vi "Test-Left Motors.vi"() -> ()   [LabVIEW 2014, in "Comp Driver.lvlib"]
uses:
  Comp Driver.lvlib
  Robot Actor Framework/Trace/Trace Controller Class/Config.ctl
  Comp Motors with Encoders/Comp Motors with Encoders Class/Motor Controller Config.ctl
  Robot/Motor with Encoders/Motors with Encoders Class/Motors with Encoders Config.ctl
  Comp Motors with Encoders/Comp Motors with Encoders Class/Encoder Config.ctl
  Comp Trace Controller/Comp Trace Controller Class/Comp Trace Controller.lvclass
  Comp Motors with Encoders/Comp Motors with Encoders Class/Comp Motors with Encoders.lvclass
  Comp Pressure/Comp Pressure Class/Comp Pressure.lvclass
  <vilib>/Rock Robotics/WPI/DriverStation/WPI_DriverStationRobotMode2.ctl
  Robot/Motor with Encoders/Motors with Encoders Messages/Set Rate Msg/Set Rate  (RPM) Msg.lvclass/Set Rate  (RPM) Msg.ctl
  <vilib>/ActorFramework/Message Enqueuer/Message Enqueuer.lvclass/Message Enqueuer.ctl
  <vilib>/ActorFramework/Message Enqueuer/Enqueue.vi
  <vilib>/ActorFramework/Message Priority Queue/Priority Enqueue.vi
  Robot/Motor with Encoders/Motors with Encoders Messages/Set Rate Msg/Set Rate  (RPM) Msg.lvclass
  <vilib>/ActorFramework/Stop Msg/Stop Msg.lvclass
  <vilib>/ActorFramework/Actor/Actor.lvclass
  Robot Actor Framework/Trace/Trace Controller Class/Trace Controller.lvclass
  Robot/Motor with Encoders/Motors with Encoders Class/Motors with Encoders.lvclass
panel:
  in  "Encoder Config":T1={"P"=1.0, "D"=0.0, "F"=0.01, "I"=0.01, "Reverse Feedback Sensor"=FALSE, "Encoder Codes Per Rev"=256}
  out "Enable Tele":bool caption="Enabled Teleop"
  in  "Stop Test Loop 1":bool=TRUE
  in  "Finish Test":bool=TRUE
  in  "Start Test":bool=TRUE
  in  "Rate (RPM)":dbl
  in  "Motos with Encoder Config":T2={"Counts  Per Revolution"=256, "Invert Encoder Direction"=FALSE, "Diameter of Revolution"=6.0, "Max RPM"=0.0, "Encoder Control"=TRUE}
  in  "Slave Motor Controller Configs":T3[](array[typedef])=[{"Device Number"=10, "Invert Motor"=FALSE}]
  in  "Master Motor Controller Config":T3={"Device Number"=9, "Invert Motor"=FALSE}
  in  "Config":T4={"Folder Pattern"="/media/sd%s1", "Starting Letter Position"=1, "Min Free Space (MB)"=50.0, "Max Folders to Check"=10, "Trace Level"=enum."Debug"} {"Min Free Space (MB)" format="%#_13g"}
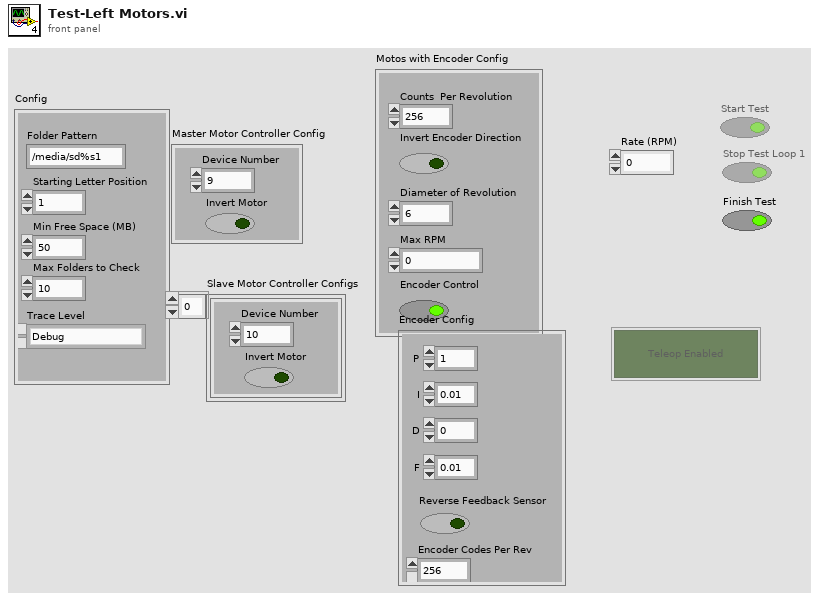
[diagram p1: front panel]
types:
  T1 = typedef "Comp Motors with Encoders.lvlib/Comp Motors with Encoders.lvclass/Encoder Config.ctl" = cluster{"P":dbl, "D":dbl, "F":dbl, "I":dbl, "Reverse Feedback Sensor":bool, "Encoder Codes Per Rev":u16}
  T2 = typedef "Motors with Encoders.lvlib/Motors with Encoders.lvclass/Motors with Encoders Config.ctl" = cluster{"Counts  Per Revolution":u32, "Invert Encoder Direction":bool, "Diameter of Revolution":dbl, "Max RPM":dbl, "Encoder Control":bool}
  T3 = typedef "Comp Motors with Encoders.lvlib/Comp Motors with Encoders.lvclass/Motor Controller Config.ctl" = cluster{"Device Number":u8, "Invert Motor":bool}
  T4 = typedef "Robot Actor Framework.lvlib/Trace.lvlib/Trace Controller.lvclass/Config.ctl" = cluster{"Folder Pattern":string, "Starting Letter Position":i32, "Min Free Space (MB)":dbl, "Max Folders to Check":u32, "Trace Level":enum16{"Critical", "Error", "Warning", "Informational", "Debug"}}
  T5 = enum8{"Enabled", "Disabled", "Disabled and Grayed Out"}
  T6 = enum16{"Critical", "Error", "Warning", "Informational", "Debug"}
  T7 = typedef "WPI_DriverStationRobotMode2.ctl" = enum16{"Autonomous Disabled", "Autonomous Enabled", "Teleop Disabled", "Teleop Enabled", "Disconnected", "Finish", "Test Disabled", "Test Enabled", "Emergency Stopped"}
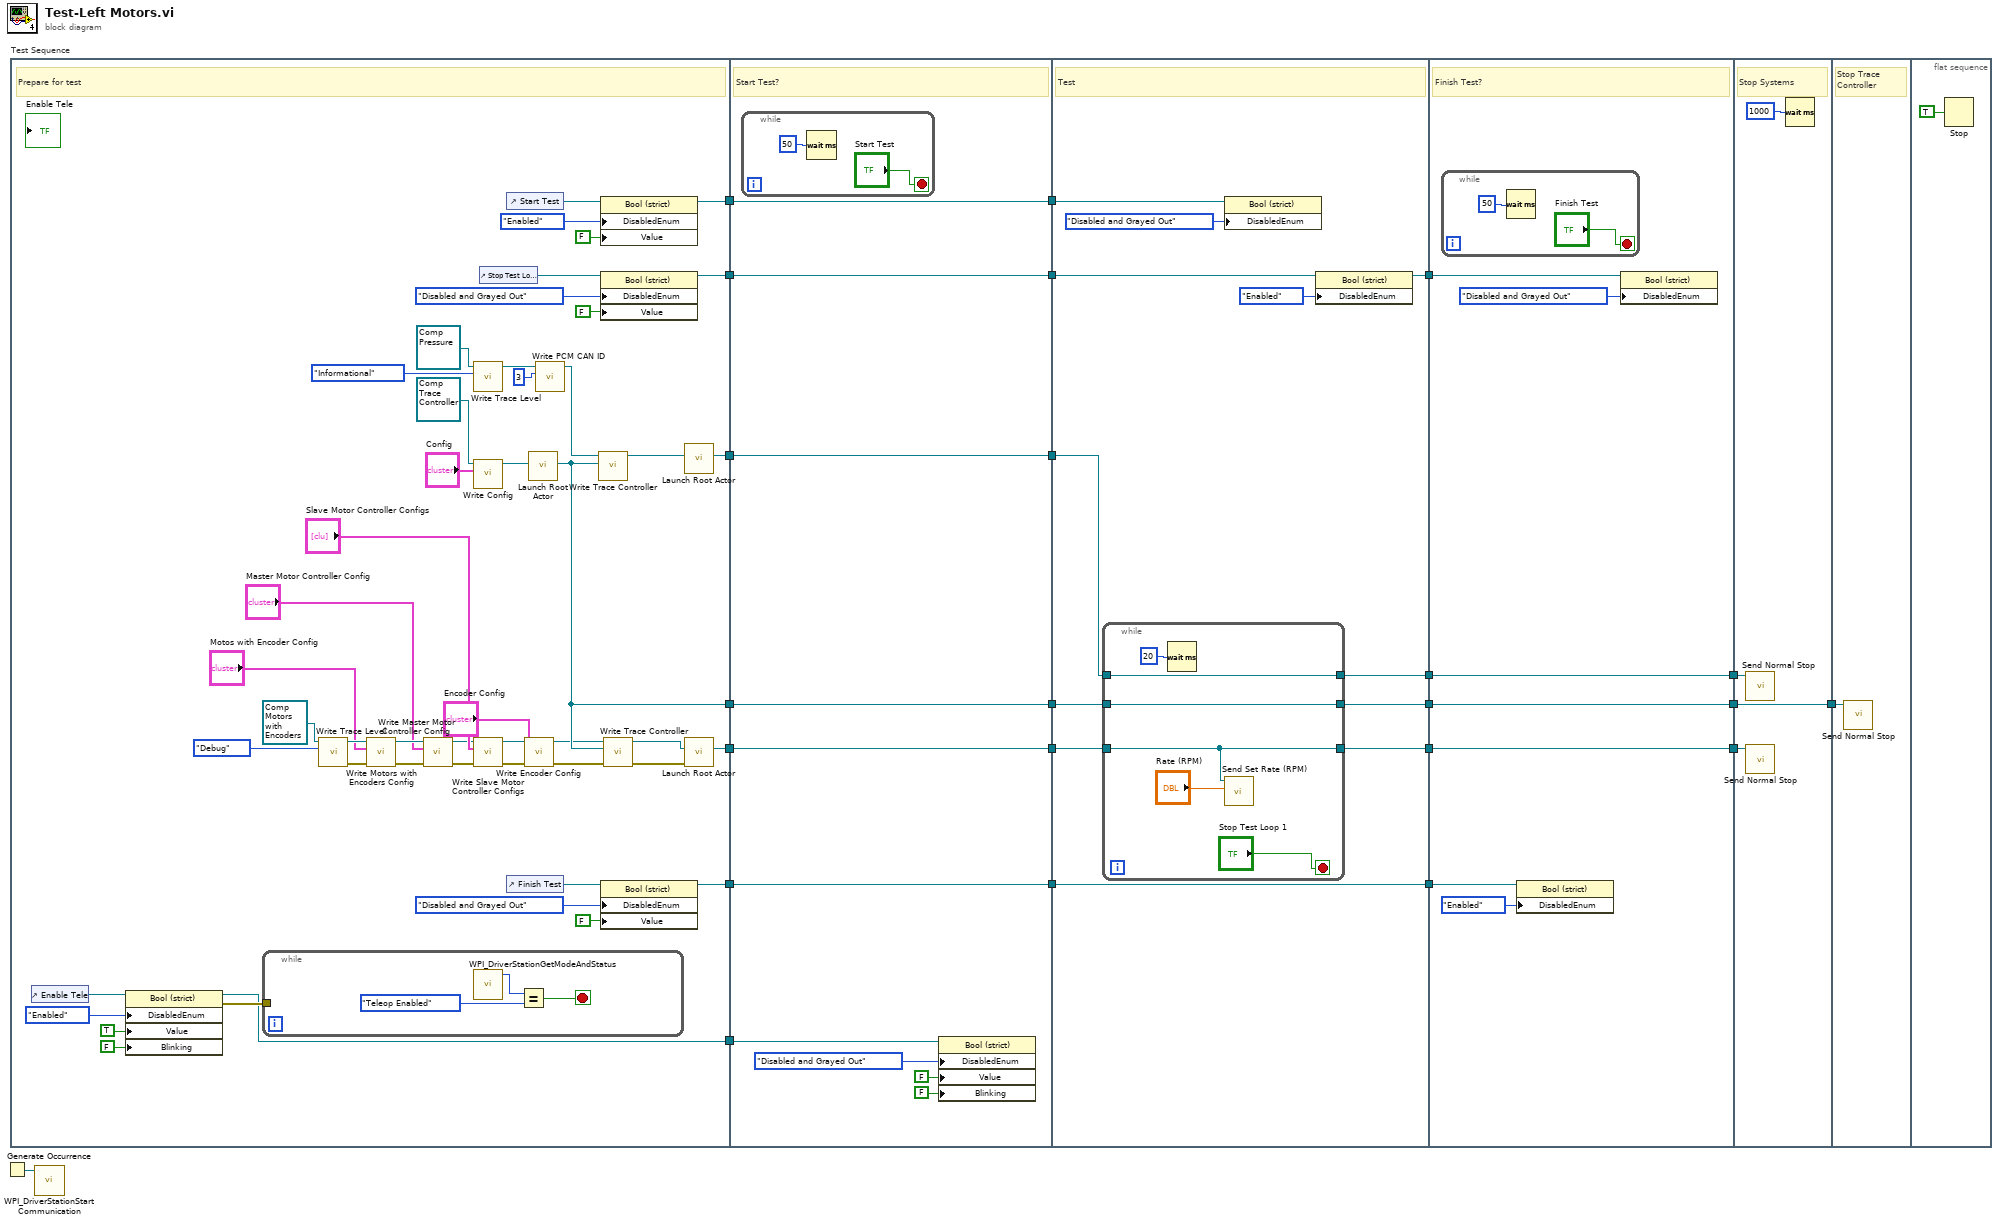
[diagram p0: block diagram]
diagram:
  n1 = Generate Occurrence() -> (w23:refnum<k4>)
  n2 = flat-sequence "Test Sequence" {
    tunnel: [w47] -> w12
    tunnel: [w49] -> w11
    tunnel: [w48] -> w10
    tunnel: [w37] -> w9
    tunnel: [w36] -> w7
    tunnel: [w35] -> w2
    tunnel: [w29] -> w1
    tunnel: [w84] -> w15
    tunnel: [w83] -> w14
    tunnel: [w82] -> w13
    tunnel: w12 -> [w84]
    tunnel: w11 -> [w83]
    tunnel: w10 -> [w82]
    tunnel: w9 -> [w81]
    tunnel: [w81] -> w8
    tunnel: w7 -> [w80]
    tunnel: [w80] -> w6
    tunnel: [w79] -> w3
    tunnel: w2 -> [w79]
    tunnel: w1 -> [w78]
    tunnel: [w93] -> w18
    tunnel: [w95] -> w17
    tunnel: [w94] -> w16
    tunnel: w15 -> [w98]
    tunnel: w14 -> [w96]
    tunnel: w13 -> [w97]
    tunnel: w8 -> [w92]
    tunnel: w6 -> [w90]
    tunnel: [w88] -> w5
    tunnel: [w87] -> w4
    tunnel: w3 -> [w87]
    tunnel: [w111] -> w21
    tunnel: [w110] -> w20
    tunnel: [w109] -> w19
    tunnel: w18 -> [w111]
    tunnel: w17 -> [w110]
    tunnel: w16 -> [w109]
    tunnel: w5 -> [w108]
    tunnel: w4 -> [w105]
    tunnel: [w117] -> w22
    tunnel: w21 -> [w117]
    tunnel: w20 -> [w116]
    tunnel: w19 -> [w114]
    tunnel: w22 -> [w118]
    frame #0 {
      # "Prepare for test"
      n3 = control-ref of="Enable Tele"() -> (w34:refnum<vi>)
      n4 = property class="Bool (strict)"(reference=w34, "DisabledEnum"=T5."Enabled" ("Disabled"), "Value"=TRUE, "Blinking"=FALSE) -> (reference out=w29:refnum<vi>, error out=w31:errorcluster)  [unwired: 1 in]
      n5 = while {
        tunnel: w31 -> [_]
        stop <- w72 stop-if-true
        n6 = call <vilib>:"WPI_DriverStationGetModeAndStatus.vi"() -> ("Robot Mode"=w74:T7)  [unwired: 10 in, 1 out]
        n7 = Equal?(x=w74, y=WPI_DriverStationRobotMode2."Teleop Enabled") -> (x = y?=w72:bool)
      }
      n8 = call-dynamic "Write Trace Level.vi"("Trace Level"=T6."Debug", "System Actor in"=refnum<class "Comp Motors with Encoders.lvclass"> refnum ("Comp Motors with Encoders.lvlib:Comp Motors with Encoders.lvclass")) -> ("error out"=w64:errorcluster, "System Actor out"=w63:refnum<class "Comp Motors with Encoders.lvclass">)  [unwired: 8 in]
      n9 = call-dynamic "Write Motors with Encoders Config.vi"("error in (no error)"=w64, "Motors with Encoders Config"="Motos with Encoder Config", "Motors with Encoders in"=w63) -> ("error out"=w58:errorcluster, "Motors with Encoders out"=w56:refnum<class "Comp Motors with Encoders.lvclass">)  [unwired: 7 in]
      n10 = call-dynamic "Write Master Motor Controller Config.vi"("error in (no error)"=w58, "Master Motor Controller Config"="Master Motor Controller Config", "Comp Motors with Encoders in"=w56) -> ("error out"=w59:errorcluster, "Comp Motors with Encoders out"=w53:refnum<class "Comp Motors with Encoders.lvclass">)  [unwired: 7 in]
      n11 = call-dynamic "Write Trace Level.vi"("Trace Level"=T6."Informational", "System Actor in"=refnum<class "Comp Pressure.lvclass"> refnum ("Comp Pressure.lvlib:Comp Pressure.lvclass")) -> ("System Actor out"=w68:refnum<class "Comp Pressure.lvclass">)  [unwired: 8 in, 1 out]
      n12 = call-dynamic "Write Config.vi"("Config"="Config", "Trace Controller in"=refnum<class "Comp Trace Controller.lvclass"> refnum ("Comp Trace Controller.lvlib:Comp Trace Controller.lvclass")) -> ("Trace Controller out"=w52:refnum<class "Comp Trace Controller.lvclass">)  [unwired: 8 in, 1 out]
      n13 = call-dynamic "Write Slave Motor Controller Configs.vi"("error in (no error)"=w59, "Slave Motor Controller Configs"="Slave Motor Controller Configs", "Comp Motors with Encoders in"=w53) -> ("error out"=w26:errorcluster, "Comp Motors with Encoders out"=w28:refnum<class "Comp Motors with Encoders.lvclass">)  [unwired: 7 in]
      n14 = control-ref of="Stop Test Loop 1"() -> (w41:refnum<vi>)
      n15 = control-ref of="Start Test"() -> (w46:refnum<vi>)
      n16 = control-ref of="Finish Test"() -> (w40:refnum<vi>)
      n17 = call-dynamic "Write Encoder Config.vi"("error in (no error)"=w26, "Encoder Config"="Encoder Config", "Comp Motors with Encoders in"=w28) -> ("error out"=w25:errorcluster, "Comp Motors with Encoders out"=w27:refnum<class "Comp Motors with Encoders.lvclass">)  [unwired: 7 in]
      n18 = call <vilib>:"Launch Root Actor.vi"("Actor"=w52) -> ("Actor's Enqueuer"=w48:refnum<class "Message Enqueuer.lvclass">)  [unwired: 9 in, 1 out]
      n19 = call-dynamic "Write PCM CAN ID.vi"("PCM CAN ID"=u8 3, "Comp Pressure in"=w68) -> ("Comp Pressure out"=w70:refnum<class "Comp Pressure.lvclass">)  [unwired: 8 in, 1 out]
      n20 = call-dynamic "Write Trace Controller.vi"("Trace Controller"=w48, "System Actor in"=w70) -> ("System Actor out"=w71:refnum<class "Comp Pressure.lvclass">)  [unwired: 8 in, 1 out]
      n21 = property class="Bool (strict)"(reference=w46, "DisabledEnum"=T5."Enabled" ("Disabled"), "Value"=FALSE) -> (reference out=w37:refnum<vi>)  [unwired: 1 in, 1 out]
      n22 = property class="Bool (strict)"(reference=w41, "DisabledEnum"=T5."Disabled and Grayed Out" ("Disabled"), "Value"=FALSE) -> (reference out=w36:refnum<vi>)  [unwired: 1 in, 1 out]
      n23 = property class="Bool (strict)"(reference=w40, "DisabledEnum"=T5."Disabled and Grayed Out" ("Disabled"), "Value"=FALSE) -> (reference out=w35:refnum<vi>)  [unwired: 1 in, 1 out]
      n24 = call-dynamic "Write Trace Controller.vi"("error in (no error)"=w25, "Trace Controller"=w48, "System Actor in"=w27) -> ("error out"=w61:errorcluster, "System Actor out"=w60:refnum<class "Comp Motors with Encoders.lvclass">)  [unwired: 7 in]
      n25 = call <vilib>:"Launch Root Actor.vi"("Actor"=w71) -> ("Actor's Enqueuer"=w49:refnum<class "Message Enqueuer.lvclass">)  [unwired: 9 in, 1 out]
      n26 = call <vilib>:"Launch Root Actor.vi"("error in (no error)"=w61, "Actor"=w60) -> ("Actor's Enqueuer"=w47:refnum<class "Message Enqueuer.lvclass">)  [unwired: 8 in, 1 out]
    }
    frame #1 {
      # "Start Test?"
      n27 = while {
        stop <- "Start Test" stop-if-true
        n28 = Wait (ms)(milliseconds to wait=u32 50) -> ()  [unwired: 1 out]
      }
      n29 = property class="Bool (strict)"(reference=w78, "DisabledEnum"=T5."Disabled and Grayed Out" ("Disabled"), "Value"=FALSE, "Blinking"=FALSE) -> ()  [unwired: 1 in, 2 out]
    }
    frame #2 {
      # "Test"
      n30 = while {
        tunnel: w97 -> [w103]
        tunnel: [w103] -> w93
        tunnel: w98 -> [w101]
        tunnel: [w101] -> w95
        tunnel: w96 -> [w100]
        tunnel: [w100] -> w94
        stop <- "Stop Test Loop 1" stop-if-true
        n31 = Wait (ms)(milliseconds to wait=u32 20) -> ()  [unwired: 1 out]
        n32 = call "Send Set Rate (RPM).vi"("Rate (RPM)"="Rate (RPM)", "Message Enqueuer"=w101) -> ()  [unwired: 8 in, 2 out]
      }
      n33 = property class="Bool (strict)"(reference=w92, "DisabledEnum"=T5."Disabled and Grayed Out" ("Disabled")) -> ()  [unwired: 1 in, 2 out]
      n34 = property class="Bool (strict)"(reference=w90, "DisabledEnum"=T5."Enabled" ("Disabled")) -> (reference out=w88:refnum<vi>)  [unwired: 1 in, 1 out]
    }
    frame #3 {
      # "Finish Test?"
      n35 = while {
        stop <- "Finish Test" stop-if-true
        n36 = Wait (ms)(milliseconds to wait=u32 50) -> ()  [unwired: 1 out]
      }
      n37 = property class="Bool (strict)"(reference=w105, "DisabledEnum"=T5."Enabled" ("Disabled")) -> ()  [unwired: 1 in, 2 out]
      n38 = property class="Bool (strict)"(reference=w108, "DisabledEnum"=T5."Disabled and Grayed Out" ("Disabled")) -> ()  [unwired: 1 in, 2 out]
    }
    frame #4 {
      # "Stop Systems"
      n39 = call <vilib>:"Send Normal Stop.vi"("Message Enqueuer"=w114) -> ()  [unwired: 10 in, 1 out]
      n40 = call <vilib>:"Send Normal Stop.vi"("Message Enqueuer"=w116) -> ()  [unwired: 10 in, 1 out]
      n41 = Wait (ms)(milliseconds to wait=u32 1000) -> ()  [unwired: 1 out]
    }
    frame #5 {
      # "Stop Trace Controller"
      n42 = call <vilib>:"Send Normal Stop.vi"("Message Enqueuer"=w118) -> ()  [unwired: 10 in, 1 out]
    }
    frame #6 {
      n43 = Stop(stop? (T)=TRUE) -> ()
    }
  }
  n44 = call <vilib>:"WPI_DriverStationStart Communication.vi"("occurrence"=w23) -> ()  [unwired: 1 in, 10 out]
